vi "Check String Type 2.vi"(8 "error in (no error)":errorcluster, 10 "String":string, 11 "Numeric Value in":refnum<class "Numeric Value.lvclass">) -> (0 "error out":errorcluster, 3 "Numeric Value out":refnum<class "Numeric Value.lvclass">)   [LabVIEW 2020]
uses:
  Value Type/Value Type.lvclass
  Numeric Value/Numeric Value.lvclass
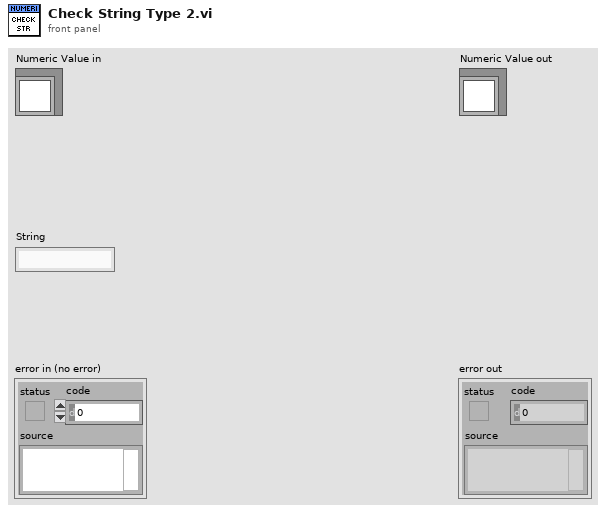
[diagram p1: front panel]
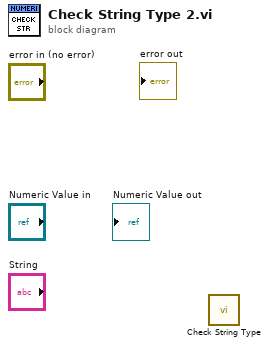
[diagram p0: block diagram]
diagram:
  n1 = call-dynamic "Check String Type.vi"() -> ()  [unwired: 10 in, 2 out]
